vi "Create.vi"(6 "Timeout ms (60000)":i32=60000, 8 "error in (no error)":errorcluster, 9 "Service Name (\"\":localhost)":string, 10 "Port(0:Ignored)":u16, 11 "Project Name (\"\": ThisApplication)":string) -> (0 "error out":errorcluster, 3 "Application out":refnum<class "Application.lvclass">)   [LabVIEW 2016, in "Application.lvclass"]
uses:
  Application.lvclass
  Application.lvclass/Application.ctl
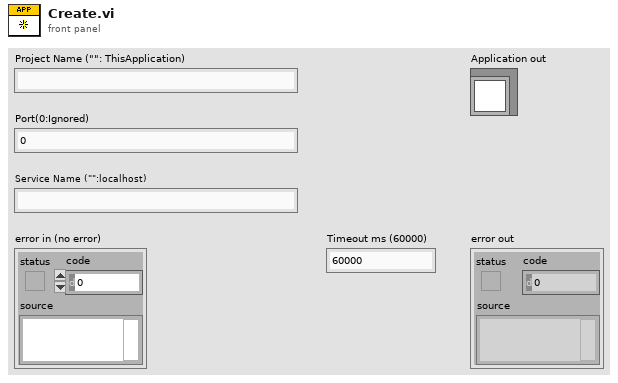
[diagram p1: front panel]
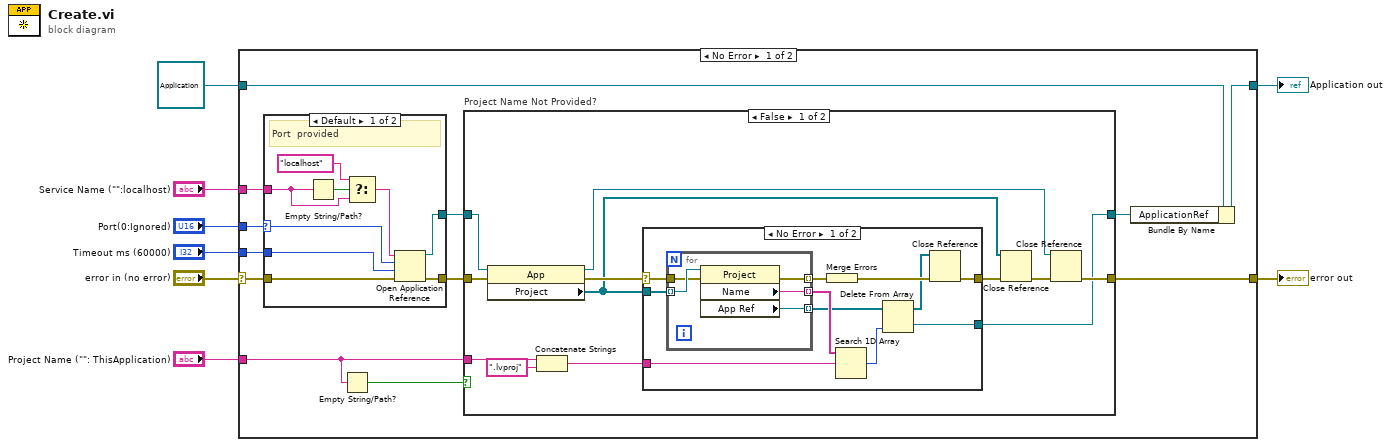
[diagram p0: block diagram]
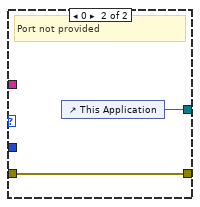
[diagram p4: hidden frame]
diagram:
  n1 = case shown="No Error" "error in (no error)" {
    selector: "error in (no error)" -> [w11 w64]
    tunnel: [w17 w64] -> w7
    tunnel: [w10 w63] -> w6
    tunnel: refnum<class "Application.lvclass"> refnum ("Application in") -> [w20 w63]
    tunnel: "Service Name (\"\":localhost)" -> [w15 _]
    tunnel: "Port(0:Ignored)" -> [w14 _]
    tunnel: "Project Name (\"\": ThisApplication)" -> [w13 _]
    tunnel: "Timeout ms (60000)" -> [w12 _]
    frame No Error {
      n2 = case shown="Default" w14 {
        selector: w14 -> [w60 _]
        tunnel: w12 -> [w59 _]
        tunnel: w11 -> [w58 w62]
        tunnel: [w53 w62] -> w18
        tunnel: w15 -> [w56 _]
        tunnel: [w52 w61] -> w16
        frame Default {
          # "Port  provided"
          n3 = Empty String/Path?(string/path=w56) -> (empty?=w57:bool)
          n4 = Select(t="localhost", s=w57, f=w56) -> (s? t:f=w54:string)
          n5 = Open Application Reference(8:w58, 9:w59, 10:w60, 11:w54) -> (0:w53:errorcluster, 3:w52:refnum<vi>)
        }
        frame 0 {
          # "Port not provided"
          n6 = control-ref of="This Application"() -> (w61:refnum<vi>)
        }
      }
      n7 = Empty String/Path?(string/path=w13) -> (empty?=w19:bool)
      n8 = case "Project Name Not Provided?" shown="False" w19 {
        tunnel: w13 -> [w26 _]
        tunnel: w18 -> [w31 w51]
        tunnel: [w32 w51] -> w17
        tunnel: [w29 w50] -> w9
        tunnel: w16 -> [w28 w50]
        frame False {
          n9 = property class="App"(reference=w28, error in=w31) -> (reference out=w27:refnum<vi>, error out=w25:errorcluster, "Project"=w23:refnum<vi>[])
          n10 = Concatenate Strings(w26, ".lvproj" ("string")) -> (w22:string)
          n11 = case shown="No Error" w25 {
            selector: w25 -> [w42 w49]
            tunnel: w23 -> [w43 _]
            tunnel: [w35 w49] -> w24
            tunnel: w22 -> [w40 _]
            tunnel: [w33 _] -> w29
            frame No Error {
              n12 = for {
                tunnel: w43 -> [w48] mode=indexing
                tunnel: w42 -> [w47]
                tunnel: [w46] -> w39 mode=indexing
                tunnel: [w45] -> w41 mode=indexing
                tunnel: [w44] -> w38 mode=indexing
                n13 = property class="Project"(reference=w48, error in=w47) -> (error out=w44:errorcluster, "Name"=w45:string, "App Ref"=w46:refnum<vi>)  [unwired: 1 out]
              }
              n14 = Merge Errors(w38) -> (w37:errorcluster)
              n15 = Search 1D Array(1D array=w41, element=w40) -> (index of element=w36:i32)  [unwired: 1 in]
              n16 = Delete From Array(array=w39, index=w36) -> (deleted portion=w33:refnum<vi>, array with subset deleted=w34:refnum<vi>[])  [unwired: 1 in]
              n17 = Close Reference(reference=w34, error in (no error)=w37) -> (error out=w35:errorcluster)
            }
            frame Error {
            }
          }
          n18 = Close Reference(reference=w23, error in (no error)=w24) -> (error out=w30:errorcluster)
          n19 = Close Reference(reference=w27, error in (no error)=w30) -> (error out=w32:errorcluster)
        }
        frame True {
        }
      }
      n20 = Bundle By Name(cluster=w20, "ApplicationRef"=w9) -> (w10:refnum<class "Application.lvclass">)
    }
    frame Error {
    }
  }
  "error out" <- w7
  "Application out" <- w6
